vi "TCP read example.vi"() -> ()   [LabVIEW 2020]
panel:
  out "Waveform Chart":u32(graph)
  out "read time":u32
  in  "stop":bool
  out "variable value":string
  out "error out":errorcluster
  out "timed out":bool
  in  "Variable name":string
  in  "Device name":string
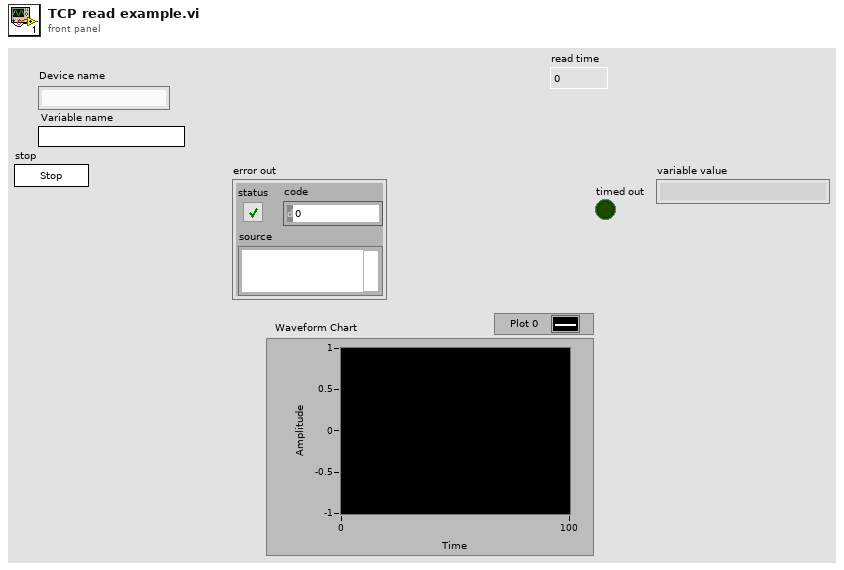
[diagram p1: front panel]
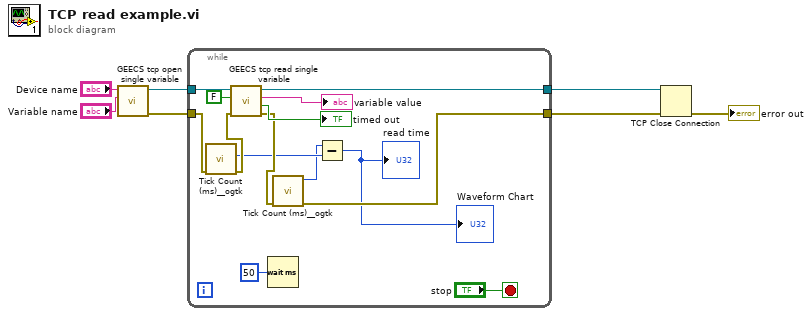
[diagram p0: block diagram]
diagram:
  n1 = call "GEECS tcp open single variable.vi"("Variable name"="Variable name", "Device name"="Device name") -> ("error out"=w3:errorcluster, "TCP Network Connection out"=w5:refnum<k5>)  [unwired: 7 in, 1 out]
  n2 = while {
    tunnel: w5 -> [w21]
    tunnel: [w20] -> w4
    tunnel: w3 -> [w14]
    tunnel: [w12] -> w2
    stop <- "stop" stop-if-true
    n3 = call <userlib>:"Tick Count (ms)__ogtk.vi"("error in (no error)"=w14) -> ("error out"=w15:errorcluster, "millisecond timer value"=w11:u32)  [unwired: 9 in]
    n4 = call "GEECS tcp read single variable.vi"("error in (no error)"=w15, "clear buffer after read"=FALSE, "TCP Network Connection in"=w21) -> ("error out"=w13:errorcluster, "timed out"=→"timed out":bool, "variable value"=→"variable value":string, "TCP Network Connection out"=w20:refnum<k5>)  [unwired: 5 in]
    n5 = Wait (ms)(milliseconds to wait=u32 50) -> ()  [unwired: 1 out]
    n6 = call <userlib>:"Tick Count (ms)__ogtk.vi"("error in (no error)"=w13) -> ("error out"=w12:errorcluster, "millisecond timer value"=w10:u32)  [unwired: 9 in]
    n7 = Subtract(x=w10, y=w11) -> (x-y=→"read time" →"Waveform Chart":u32)
  }
  n8 = TCP Close Connection(connection ID=w4, error in (no error)=w2) -> (error out=→"error out":errorcluster)  [unwired: 1 in, 1 out]
